vi "Write Stop Reason.vi"(8 "error in (no error)":errorcluster, 10 "Stop Reason":T1, 11 "Iterator Actor in":refnum<class "Iterator Actor.lvclass">) -> (0 "error out":errorcluster, 3 "Iterator Actor out":refnum<class "Iterator Actor.lvclass">)   [LabVIEW 2020, in "Iterator Actor.lvlib" / "Iterator Actor.lvclass"]
uses:
  Iterator Actor.lvclass
  Iterator Actor.lvclass/Iterator Actor.ctl
  Stop Reason.ctl
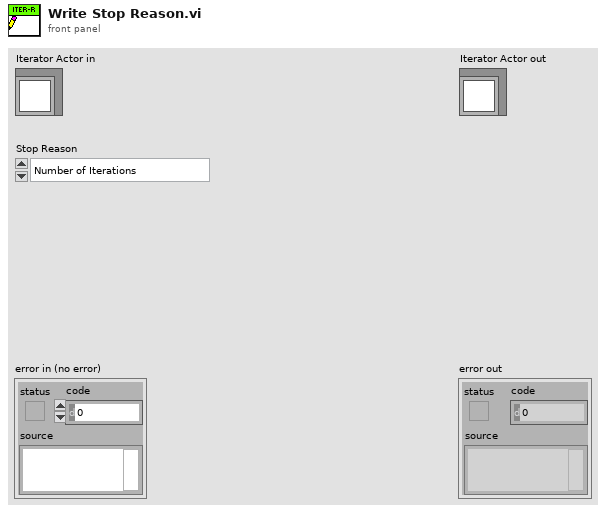
[diagram p1: front panel]
types:
  T1 = typedef "Iterator Actor.lvlib/Iterator Actor.lvclass/Stop Reason.ctl" = enum16{"Number of Iterations", "Time Elapsed", "Stopped Internally", "Stopped Externally"}
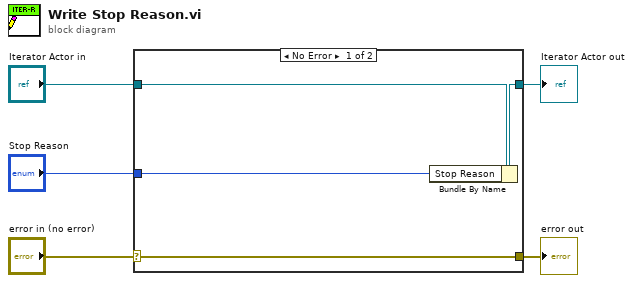
[diagram p0: block diagram]
diagram:
  n1 = case shown="No Error" "error in (no error)" {
    selector: "error in (no error)" -> [w9 w10]
    tunnel: [w9 w10] -> w4
    tunnel: [w7 w11] -> w2
    tunnel: "Iterator Actor in" -> [w8 w11]
    tunnel: "Stop Reason" -> [w6 _]
    frame No Error {
      n2 = Bundle By Name(cluster=w8, "Stop Reason"=w6) -> (w7:refnum<class "Iterator Actor.lvclass">)
    }
    frame Error {
    }
  }
  "error out" <- w4
  "Iterator Actor out" <- w2
